vi "OctaveBandsProcess.vi"(0 "averaging type":T2(ring)=enum."Exponential", 5 "data":waveform(dbl), 7 "dB On (T)":bool) -> (2 "filter settled":bool, 3 "nominal frequencies [Hz]":dbl[](array[numeric]), 4 "frequency range":T3={"low band"=enum."20 Hz", "high band"=enum."20000 Hz"}, 6 "band power":dbl[](array[numeric]), 10 "octave spectrum":T1, 12 "dB On":bool=TRUE, 13 "unit label":string, 14 "total band power":dbl)   [LabVIEW 2017]
uses:
  <vilib>/addons/Sound and Vibration/svt_Octave/SoundVib_Octave_2014 standard.lvlib
  <vilib>/addons/Sound and Vibration/svt_Calibration/SoundVib_Calibration.lvlib
  <vilib>/addons/Sound and Vibration/svt_Calibration/SVL Scale Voltage to EU (1 Ch).vi
  <vilib>/addons/Sound and Vibration/svt_Octave_2014 standard/SVT Third-octave Analysis (1 Ch).vi
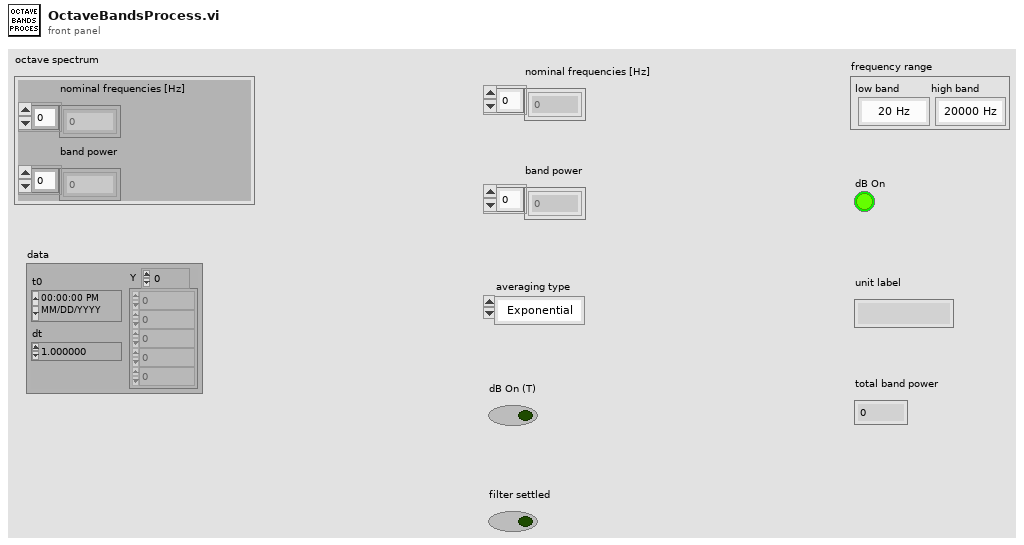
[diagram p1: front panel]
types:
  T1 = cluster{"nominal frequencies [Hz]":dbl[], "band power":dbl[]}
  T2 = enum16{"Linear", "Exponential", "Equal confidence", "Peak"}
  T3 = cluster{"low band":enum16{"20 Hz", "25 Hz", "31.5 Hz", "40 Hz", "50 Hz", "63 Hz", "80 Hz", "100 Hz", "125 Hz", "160 Hz", "200 Hz", "250 Hz", "315 Hz", "400 Hz", "500 Hz", "630 Hz", "800 Hz", "1000 Hz", "1250 Hz", "1600 Hz", "2000 Hz", "2500 Hz", "3150 Hz", "4000 Hz", "5000 Hz", "6300 Hz", "8000 Hz", "10000 Hz", "12500 Hz", "16000 Hz", "20000 Hz"}, "high band":enum16{"20 Hz", "25 Hz", "31.5 Hz", "40 Hz", "50 Hz", "63 Hz", "80 Hz", "100 Hz", "125 Hz", "160 Hz", "200 Hz", "250 Hz", "315 Hz", "400 Hz", "500 Hz", "630 Hz", "800 Hz", "1000 Hz", "1250 Hz", "1600 Hz", "2000 Hz", "2500 Hz", "3150 Hz", "4000 Hz", "5000 Hz", "6300 Hz", "8000 Hz", "10000 Hz", "12500 Hz", "16000 Hz", "20000 Hz"}}
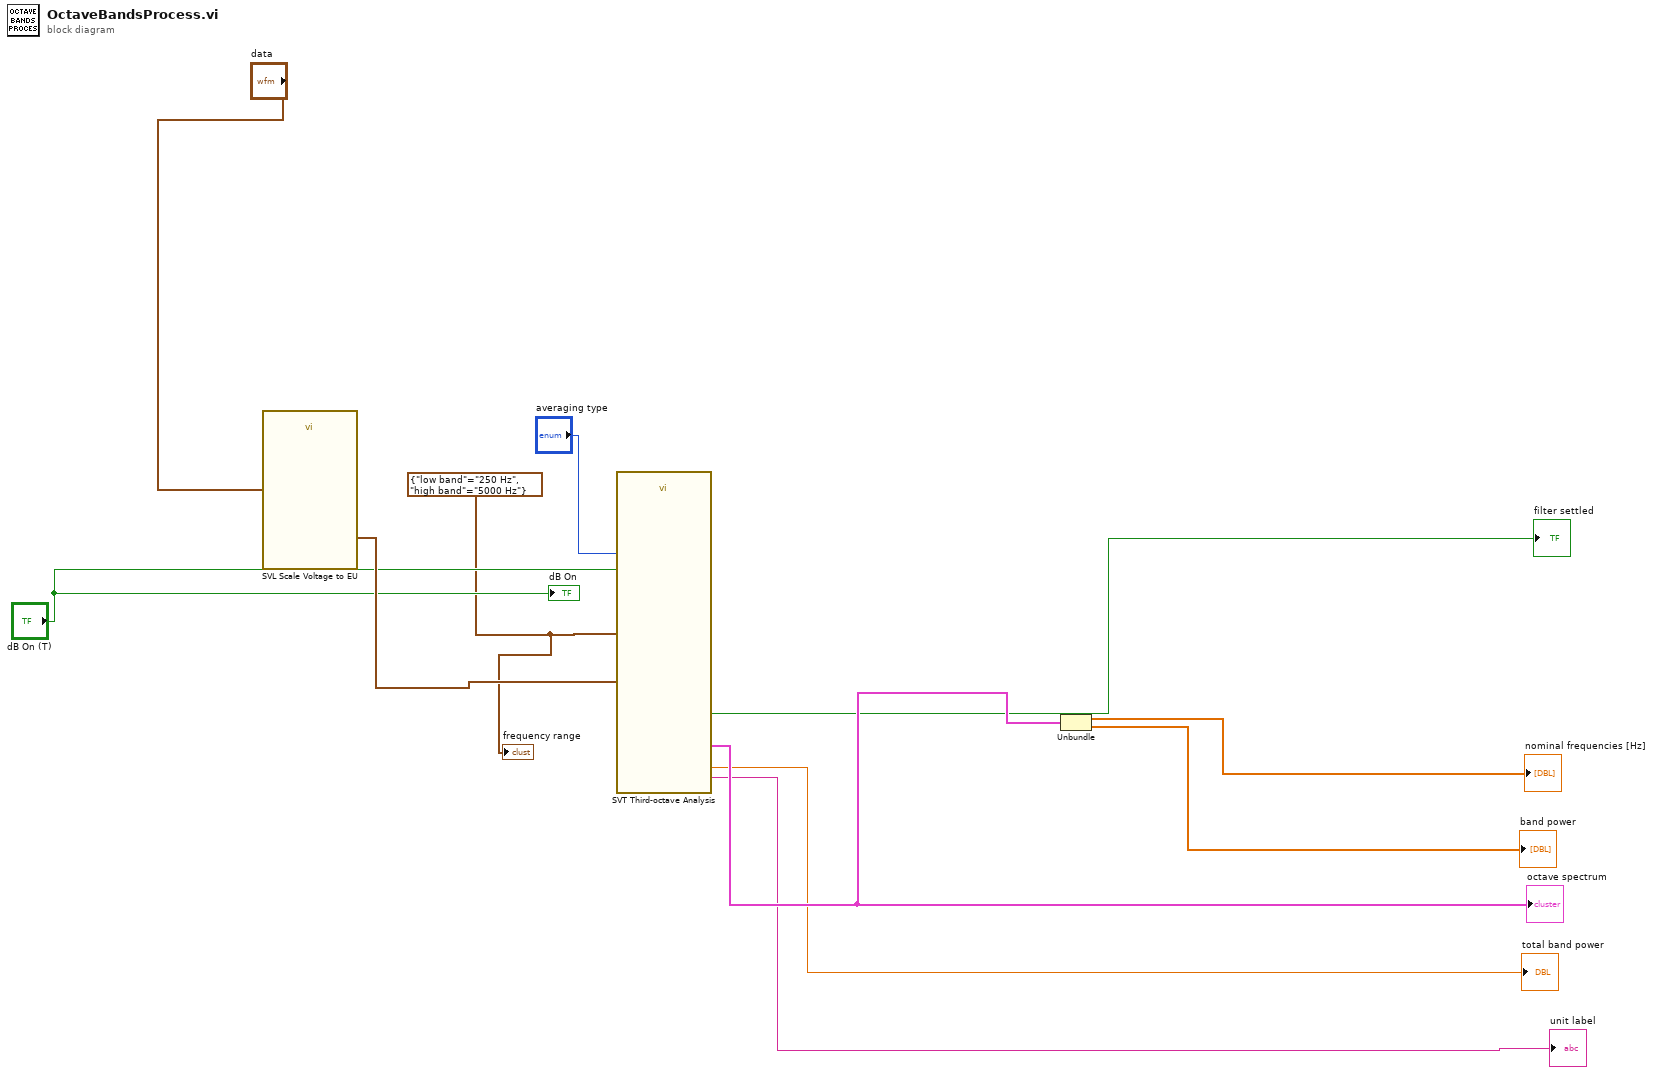
[diagram p0: block diagram]
diagram:
  w9 = T3 {"low band"=enum."250 Hz", "high band"=enum."5000 Hz"} ("frequency range")
  n1 = call-poly <vilib>:"SVL Scale Voltage to EU.vi"("signal [V]"="data") -> ("scaled signal [EU]"=w11:waveform(dbl))  [unwired: 8 in, 2 out]
  n2 = call-poly <vilib>:"SVT Third-octave Analysis.vi"("scaled signal [EU]"=w11, "frequency range"=w9, "dB On (T)"="dB On (T)", "averaging type"="averaging type") -> ("filter settled"=→"filter settled":bool, "octave spectrum"=w8:T1, "unit label"=→"unit label":string, "total band power"=→"total band power":dbl)  [unwired: 6 in, 2 out]
  "octave spectrum" <- w8
  n3 = Unbundle(w8) -> ("nominal frequencies [Hz]"=→"nominal frequencies [Hz]":dbl[], "band power"=→"band power":dbl[])
  "frequency range" <- w9
  "dB On" <- "dB On (T)"
